vi "Set Resistance.vi"(0 "object in":refnum<class "HPS-17000-PowerModule.lvclass">, 5 "resistance (Ohm)":dbl, 11 "Error In":errorcluster) -> (4 "object out":refnum<class "HPS-17000-PowerModule.lvclass">, 15 "Error Out":errorcluster)   [LabVIEW 2023, in "HPS-17000-PowerModule.lvlib" / "HPS-17000-PowerModule.lvclass"]
uses:
  HPS-17000-PowerModule.lvclass
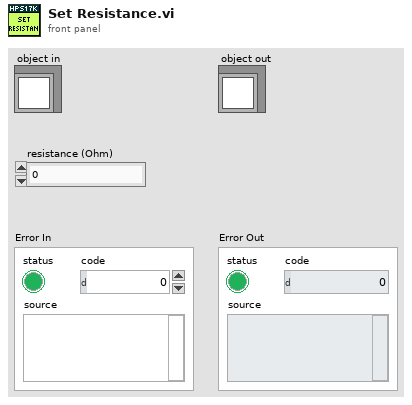
[diagram p1: front panel]
types:
  T1 = typedef "HPS-17000-PowerModule.lvlib/HPS-17000-PowerModule.lvclass/ObjectAttributes.ctl" = cluster{"HPS17000 IP Addresses":string[], "HPS Topology":enum16{"SINGLE", "MULTI"}, "GM ID":string, "TSN NIC IP Address":string, "HPS17000 Refs":refnum<class "HPS-17000.lvclass">[], "Stream Queues":refnum<queue>[], "connected":bool, "reserved":bool, "events":T2, "nibatterycycler_grpc_Setpoint":T3, "last timestamp":i64, "setpoint stream config":T4, "mode":T5, "range":T6}
  T2 = typedef "HPS-17000.lvclass/Multi-Cycler Events.ctl" = cluster{"heartbeats events":refnum<user-event>[], "faults events":refnum<user-event>[], "network sync event":refnum<user-event>[], "setpoint status event":refnum<user-event>[]}
  T3 = typedef "NI_BC_client.lvlib/nibatterycycler_grpc_Setpoint.ctl" = cluster{"voltage":sgl, "current":sgl, "min_power":sgl, "max_power":sgl, "resistance":sgl}
  T4 = typedef "Cycler.lvclass/Setpoint Stream Basic Config.ctl" = cluster{"local address":string, "receiver port":u16}
  T5 = typedef "HPS-17000-PowerModule.lvlib/HPS-17000-PowerModule.lvclass/Mode.ctl" = u16
  T6 = typedef "PowerModuleInterface.lvlibp/PowerModuleInterface.lvclass/Range.ctl" = cluster{"Current Max (A)":dbl, "Current Min (A)":dbl, "Voltage Max (V)":dbl, "Voltage Min (V)":dbl}
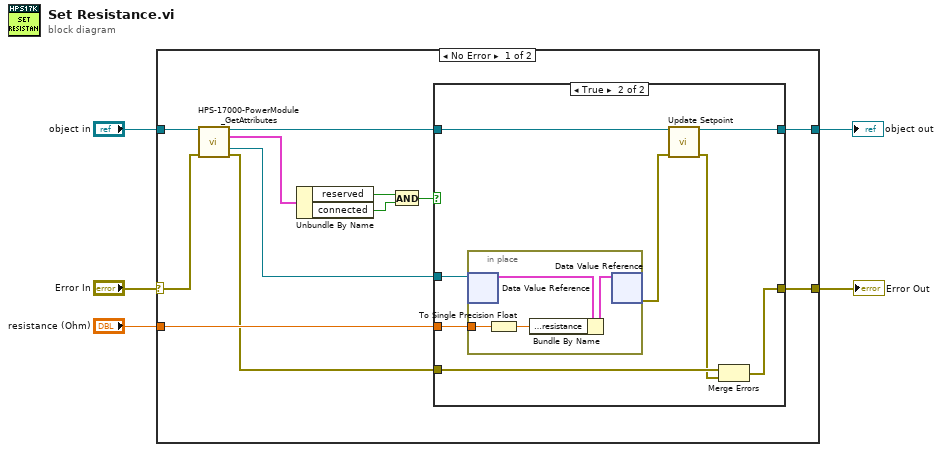
[diagram p0: block diagram]
diagram:
  n1 = case shown="No Error" "Error In" {
    selector: "Error In" -> [w16 w32]
    tunnel: "object in" -> [w17 w33]
    tunnel: [w13 w33] -> w1
    tunnel: [w12 w32] -> w2
    tunnel: "resistance (Ohm)" -> [w11 _]
    frame No Error {
      n2 = call "HPS-17000-PowerModule_GetAttributes.vi"("reference in"=w17, "Error In"=w16) -> ("reference out"=w14:refnum<class "HPS-17000-PowerModule.lvclass">, "Data"=w10:T1, "DataRef"=w15:refnum<data-value>, "Error Out"=w9:errorcluster)  [unwired: 10 in]
      n3 = Unbundle By Name(w10) -> ("reserved"=w8:bool, "connected"=w7:bool)
      n4 = And(x=w8, y=w7) -> (x .and. y?=w6:bool)
      n5 = case shown="True" w6 {
        tunnel: w15 -> [_ w27]
        tunnel: w14 -> [w19 w26]
        tunnel: [w19 w25] -> w13
        tunnel: [w18 w20] -> w12
        tunnel: w11 -> [_ w24]
        tunnel: w9 -> [w18 w23]
        frame False {
        }
        frame True {
          n6 = in-place {
            in-place-border: w24 -> [w29]
            n7 = in-place-dvr #1(w27) -> (w31:T1)  [unwired: 1 out]
            n8 = To Single Precision Float(number=w29) -> (single precision float=w28:sgl)
            n9 = Bundle By Name(cluster=w31, "nibatterycycler_grpc_Setpoint.resistance"=w28) -> (w30:T1)
            n10 = in-place-dvr #1(w30) -> (w22:errorcluster)  [unwired: 1 out]
          }
          n11 = call "Update Setpoint.vi"("reference in"=w26, "Error In"=w22) -> ("reference out"=w25:refnum<class "HPS-17000-PowerModule.lvclass">, "Error Out"=w21:errorcluster)  [unwired: 12 in]
          n12 = Merge Errors(w23, w21) -> (w20:errorcluster)
        }
      }
    }
    frame Error {
    }
  }
  "Error Out" <- w2
  "object out" <- w1
